vi "Get_Local_IP_Addres.vi"() -> (3 "IP Address":string)   [LabVIEW 2015]
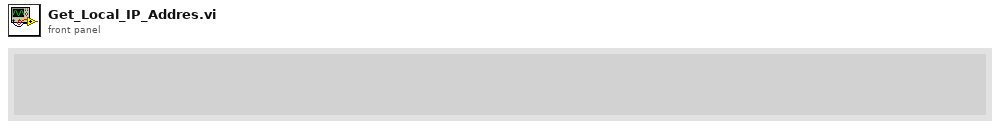
[diagram p1: front panel]
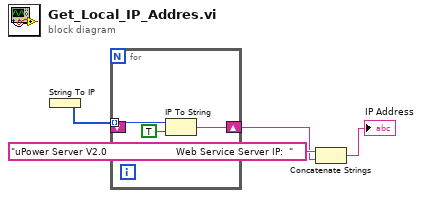
[diagram p0: block diagram]
diagram:
  n1 = String To IP() -> (0:w1:u32[])  [unwired: 1 in]
  n2 = for {
    tunnel: w1 -> [w7] mode=indexing
    shift-right: [w5] -> w2
    shift-left: _ -> [_]
    n3 = IP To String(1:TRUE ("dot notation? (F)"), 2:w7) -> (0:w5:string)
  }
  n4 = Concatenate Strings("uPower Server V2.0                       Web Service Server IP:  " ("string"), w2) -> (→"IP Address":string)
